vi "Sliders.vi"() -> ()   [LabVIEW 2010]
panel:
  in  "Slide 3":dbl(slide) scale=0.0..10.0
  in  "Slide 2":dbl(slide) scale=0.0..10.0
  in  "Slide":dbl(slide) scale=0.0..10.0
  # "Sliders"
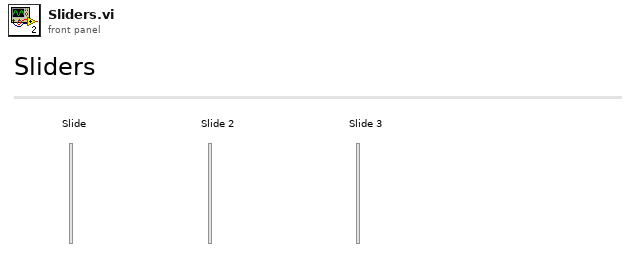
[diagram p1: front panel]
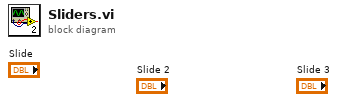
[diagram p0: block diagram]
diagram:
